vi "DrawPlannedPath.vi"(8 "error in (no error)":errorcluster, 10 "path points":cluster{"x":dbl, "y":dbl}[](array[cluster]), 11 "picture":picture) -> (0 "error out":errorcluster, 3 "new picture":picture)   [LabVIEW 2009, in "Host.lvlib" / "Draw.lvlib"]
uses:
  Draw.lvlib
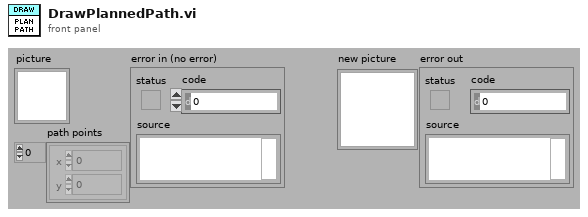
[diagram p1: front panel]
types:
  T1 = cluster{"Width":u16, "Style":enum32{"Solid", "Dash", "Dot", "DashDot", "DashDotDot"}}
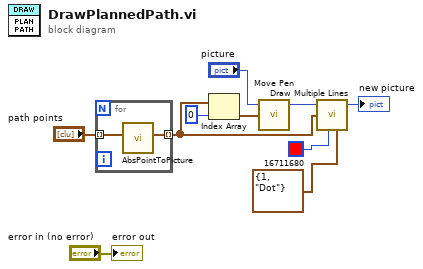
[diagram p0: block diagram]
diagram:
  n1 = for {
    tunnel: "path points" -> [w12] mode=indexing
    tunnel: [w11] -> w1 mode=indexing
    n2 = call "AbsPointToPicture.vi"("input position"=w12) -> ("output point"=w11:cluster{"x":i16, "y":i16})  [unwired: 10 in]
  }
  n3 = Index Array(array=w1, index=0) -> (element=w4:cluster{"x":i16, "y":i16})
  n4 = call <vilib>:"Move Pen.vi"("new position"=w4, "picture"="picture") -> ("new picture"=w8:picture)  [unwired: 3 in]
  n5 = call <vilib>:"Draw Multiple Lines.vi"("picture"=w8, "line endpoints"=w1, "color(black)"=u32 16711680, "pen"=T1 {"Width"=1, "Style"=enum."Dot"}) -> ("new picture"=→"new picture":picture)  [unwired: 5 in]
  "error out" <- "error in (no error)"
